vi "MCB Parser.vi"(8 "error in (no error)":errorcluster, 10 "RDS Serial Frame":refnum<class "RDS Serial Frame.lvclass">, 11 "MCB Instrument in":refnum<class "MCB Instrument.lvclass">) -> (0 "error out":errorcluster, 1 "Valid?":bool, 2 "RDS Framework.lvlib:RDS Message.lvclass":refnum<class "RDS Message.lvclass">, 3 "MCB Instrument out":refnum<class "MCB Instrument.lvclass">)   [LabVIEW 2015, in "MCB Instrument.lvlib" / "MCB Instrument.lvclass"]
uses:
  MCB Instrument.lvclass
  Libraries/RDS Framework/RDS Message Class/RDS Message.lvclass
  Libraries/RDS Serial Handler/RDS Serial Frame.lvclass
  Libraries/RDS Child Messages/MCB/MCB Channel.ctl
  Libraries/RDS Child Messages/MCB/MCB Motor Status.ctl
  Libraries/RDS Serial Handler/RDS Serial Frame.lvclass/RDS Serial Frame.ctl
  Libraries/RDS Child Messages/MCB/MCB Status Message/MCB Status.lvclass
  Libraries/RDS Framework/RDS Message ID.ctl
  MCB Instrument.lvclass/MCB Instrument.ctl
  Libraries/RDS Child Messages/MCB/MCB Status Message/MCB Status.lvclass/MCB Status.ctl
  Libraries/RDS Framework/RDS Message Class/RDS Message.lvclass/RDS Message.ctl
  Libraries/RDS Serial Handler/RDS Serial Handler.lvlib
  Libraries/RDS Child Messages/RDS Child Messages.lvlib
panel:
  out "output cluster":T1
  out "Motor":T2
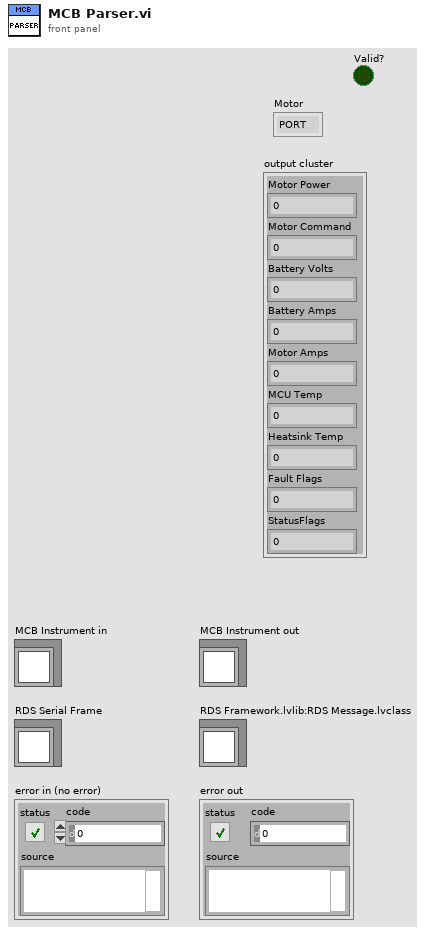
[diagram p1: front panel]
types:
  T1 = typedef "RDS Child Messages.lvlib/MCB Motor Status.ctl" = cluster{"Motor Power":i16, "Motor Command":i16, "Battery Volts":sgl, "Battery Amps":sgl, "Motor Amps":sgl, "MCU Temp":i16, "Heatsink Temp":i16, "Fault Flags":u16, "StatusFlags":u16}
  T2 = typedef "RDS Child Messages.lvlib/MCB Channel.ctl" = enum16{"PORT", "STBD"}
  T3 = typedef "RDS Child Messages.lvlib/RDS Message ID.ctl" = enum16{"RDS Hello World", "String Message", "AIP_Status", "AIP_Command", "GPS_Data", "MCB_Command", "MCB_Status", "Compass_Data", "Depth_Data", "Battery_Data", "Contoller_State", "Set_Mag_Dev", "BTB_Shutdown", "State_Sample_Request", "State_Sample", "PID_Gains_Set", "Helm_Limiter_Set", "Helm_Heading_Command", "Helm_Steering_Command", "Helm_Status", "Controller_Message", "AIP_Set_Min_Depth", "Mission_Controller_State", "Mission_Upload", "Mission_Set_Op_and_Run", "Mission_Settings_Set"}
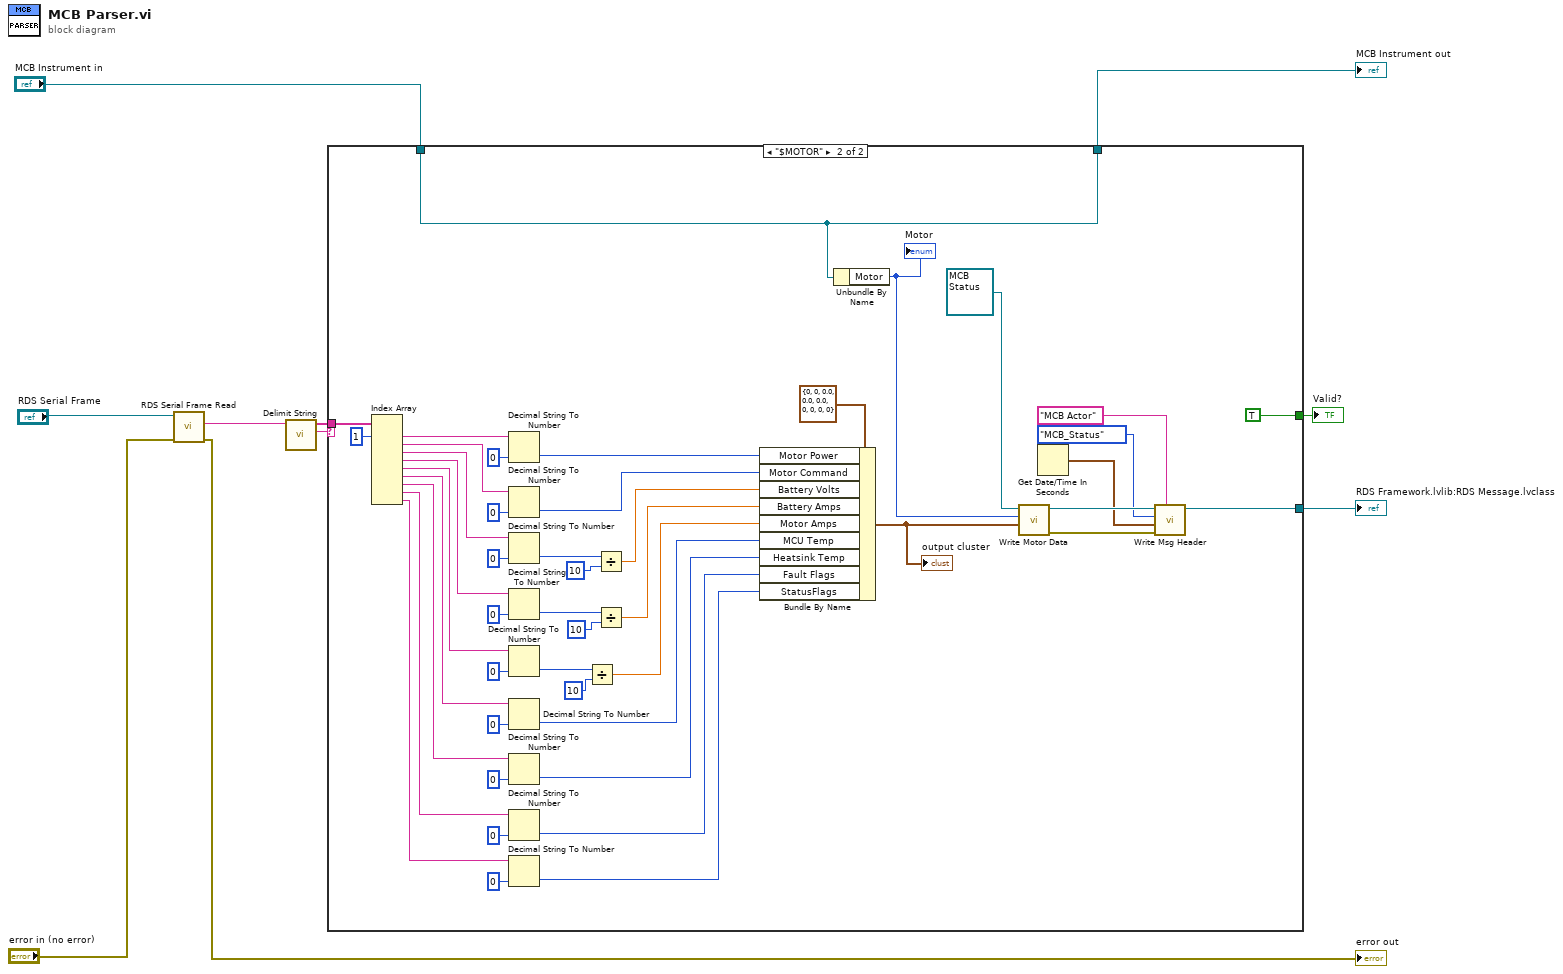
[diagram p0: block diagram]
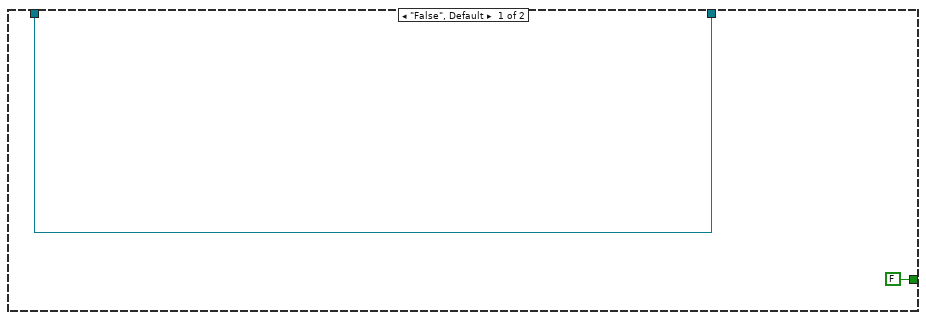
[diagram p2: hidden frame]
diagram:
  n1 = call "RDS Serial Frame Read.vi"("error in (no error)"="error in (no error)", "RDS Serial Frame in"="RDS Serial Frame") -> ("error out"=→"error out":errorcluster, "Serial String"=w4:string)  [unwired: 6 in, 2 out]
  n2 = call "Delimit String.vi"("Serial String"=w4) -> ("First Element"=w5:string, "All Elements"=w6:string[])  [unwired: 9 in]
  n3 = case shown="\"$MOTOR\"" w5 {
    tunnel: w6 -> [_ w58]
    tunnel: [w12 w56] -> w7
    tunnel: "MCB Instrument in" -> [w12 w56]
    tunnel: [_ w24] -> w2
    tunnel: [FALSE TRUE] -> w1
    frame "False", Default {
    }
    frame "$MOTOR" {
      n4 = Index Array(array=w58, index #1=1 ("index")) -> (element #1=w57:string, element #2=w53:string, element #3=w49:string, element #4=w42:string, element #5=w39:string, element #6=w36:string, element #7=w34:string, element #8=w33:string, element #9=w16:string)  [unwired: 8 in]
      n5 = Decimal String To Number(string=w57, default (0L)=i16 0 ("default (0 I32)")) -> (number=w55:i16)  [unwired: 1 in, 1 out]
      n6 = Decimal String To Number(string=w53, default (0L)=i16 0 ("default (0 I32)")) -> (number=w52:i16)  [unwired: 1 in, 1 out]
      n7 = Decimal String To Number(string=w49, default (0L)=i16 0 ("default (0 I32)")) -> (number=w48:i16)  [unwired: 1 in, 1 out]
      n8 = Decimal String To Number(string=w42, default (0L)=i16 0 ("default (0 I32)")) -> (number=w44:i16)  [unwired: 1 in, 1 out]
      n9 = Decimal String To Number(string=w39, default (0L)=i16 0 ("default (0 I32)")) -> (number=w22:i16)  [unwired: 1 in, 1 out]
      n10 = Decimal String To Number(string=w36, default (0L)=i16 0 ("default (0 I32)")) -> (number=w14:i16)  [unwired: 1 in, 1 out]
      n11 = Decimal String To Number(string=w34, default (0L)=u16 0 ("default (0 I32)")) -> (number=w20:u16)  [unwired: 1 in, 1 out]
      n12 = Decimal String To Number(string=w33, default (0L)=u16 0 ("default (0 I32)")) -> (number=w19:u16)  [unwired: 1 in, 1 out]
      n13 = Decimal String To Number(string=w16, default (0L)=u16 0 ("default (0 I32)")) -> (number=w15:u16)  [unwired: 1 in, 1 out]
      n14 = Divide(x=w22, y=i16 10) -> (x/y=w21:sgl)
      n15 = Divide(x=w48, y=i16 10) -> (x/y=w46:sgl)
      n16 = Divide(x=w44, y=i16 10) -> (x/y=w41:sgl)
      n17 = Bundle By Name(cluster=T1 {"Motor Power"=0, "Motor Command"=0, "Battery Volts"=0.0, "Battery Amps"=0.0, "Motor Amps"=0.0, "MCU Temp"=0, "Heatsink Temp"=0, "Fault Flags"=0, "StatusFlags"=0} ("Motor Data"), "Motor Power"=w55, "Motor Command"=w52, "Battery Volts"=w46, "Battery Amps"=w41, "Motor Amps"=w21, "MCU Temp"=w14, "Heatsink Temp"=w20, "Fault Flags"=w19, "StatusFlags"=w15) -> (w30:T1)
      "output cluster" <- w30
      n18 = Unbundle By Name(w56) -> ("Motor"=w31:T2)
      "Motor" <- w31
      n19 = call "Write Motor Data.vi"("Motor Data"=w30, "Motor"=w31, "MCB Status in"=refnum<class "MCB Status.lvclass"> refnum) -> ("error out"=w25:errorcluster, "MCB Status out"=w29:refnum<class "MCB Status.lvclass">)  [unwired: 7 in]
      n20 = Get Date/Time In Seconds() -> (seconds since 1Jan1904=w26:timestamp)
      n21 = call "Write Msg Header.vi"("Sender Name"="MCB Actor", "error in (no error)"=w25, "Time Stamp"=w26, "Msg ID"=RDS_Message_ID."MCB_Status", "RDS Message in"=w29) -> ("RDS Message out"=w24:refnum<class "MCB Status.lvclass">)  [unwired: 5 in, 1 out]
    }
  }
  "MCB Instrument out" <- w7
  "RDS Framework.lvlib:RDS Message.lvclass" <- w2
  "Valid?" <- w1
